vi "LCWP950 Signal Acquisition.vi"(0 "VISA resource name in":refnum<visa-resource-name>="VICP::172.25.1.26", 3 "Query Instrument?":bool=TRUE, 5 "error in (no error)":errorcluster) -> (14 "VISA resource name out":refnum<visa-resource-name>, 19 "error out":errorcluster)   [LabVIEW 2012]
uses:
  <vilib>/Instr/_visa.llb/VISA Open Access Mode.ctl
panel:
  in  "?":T1(tab)
  in  "Save Folder":path=path "C:/TEST"
  out "Run Count":i32
  in  "N Loops":i32
  out "C1:\nC2:\n   t:":string
  in  "Byte count":u32=160800
  out "Identity":string
  # "Neil McBlane 2016"
  # "NOTE: VISA Read byte count will need increased for reading >400 points - e.g. try\n320800 for 800 points. For n points: 4 bytes per point, n+2 points recorded 100 times."
  # "NOTE: code 1073676294 is not an error - it indicates the buffer has been read in its entirety"
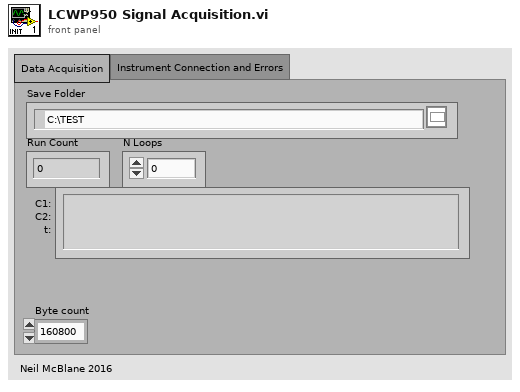
[diagram p1: front panel]
types:
  T1 = enum32{"Data Acquisition", "Instrument Connection and Errors"}
  T2 = typedef "VISA Open Access Mode.ctl" = u32
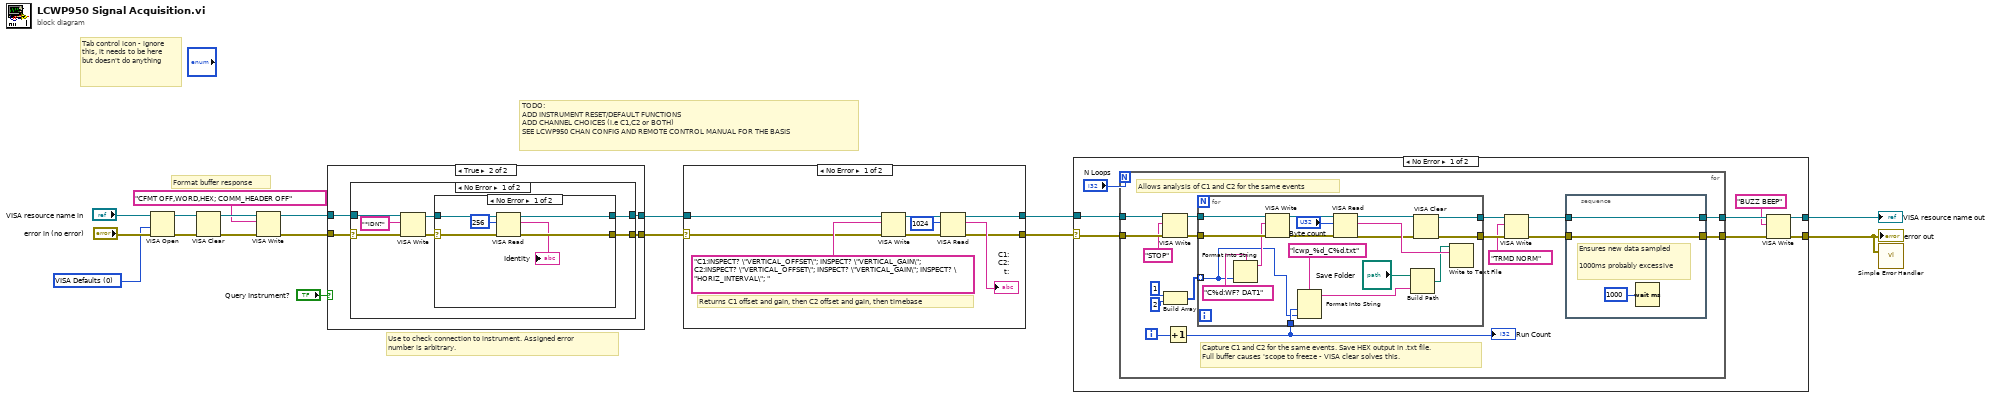
[diagram p0: block diagram]
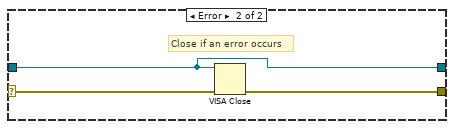
[diagram p2: hidden frame]
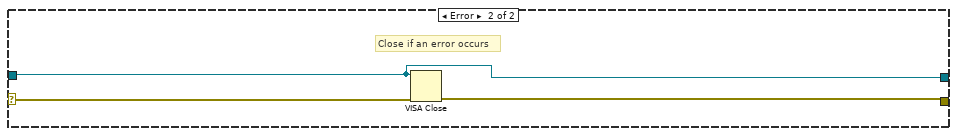
[diagram p3: hidden frame]
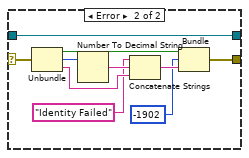
[diagram p5: hidden frame]
diagram:
  w15 = T2 0 items=["VISA Defaults"=0, "Exclusive Lock"=1, "Load Configured Settings"=4] ("Access Mode")
  # "Tab control icon - ignore this, it needs to be here but doesn't do anything"
  # "Use to check connection to instrument. Assigned error number is arbitrary."
  # "Format buffer response"
  # "TODO: \nADD INSTRUMENT RESET/DEFAULT FUNCTIONS\nADD CHANNEL CHOICES (i.e C1,C2 or BOTH)\nSEE LCWP950 CHAN CONFIG AND REMOTE CONTROL MANUAL FOR THE BASIS"
  n1 = VISA Open(access mode=w15, error in (no error)="error in (no error)", VISA resource name="VISA resource name in") -> (VISA resource name=w14:refnum<visa-resource-name>, error out=w13:errorcluster)  [unwired: 2 in]
  n2 = VISA Clear(VISA resource name=w14, error in (no error)=w13) -> (VISA resource name out=w9:refnum<visa-resource-name>, error out=w8:errorcluster)
  n3 = VISA Write(VISA resource name=w9, write buffer="CFMT OFF,WORD,HEX; COMM_HEADER OFF", error in (no error)=w8) -> (VISA resource name out=w6:refnum<visa-resource-name>, error out=w7:errorcluster)  [unwired: 1 out]
  n4 = case shown="True" "Query Instrument?" {
    tunnel: w6 -> [w19 w23]
    tunnel: w7 -> [w18 w22]
    tunnel: [w18 w21] -> w1
    tunnel: [w19 w20] -> w4
    frame False {
    }
    frame True {
      n5 = case shown="No Error" w22 {
        selector: w22 -> [w28 w48]
        tunnel: w23 -> [w29 w47]
        tunnel: [w24 w48] -> w21
        tunnel: [w26 w47] -> w20
        frame No Error {
          n6 = VISA Write(VISA resource name=w29, write buffer="*IDN?", error in (no error)=w28) -> (VISA resource name out=w27:refnum<visa-resource-name>, error out=w25:errorcluster)  [unwired: 1 out]
          n7 = case shown="No Error" w25 {
            selector: w25 -> [w36 w45]
            tunnel: w27 -> [w35 w46]
            tunnel: [w34 w46] -> w26
            tunnel: [w33 w43] -> w24
            frame No Error {
              n8 = VISA Read(VISA resource name=w35, byte count=u32 256, error in (no error)=w36) -> (VISA resource name out=w34:refnum<visa-resource-name>, read buffer=→"Identity":string, error out=w33:errorcluster)  [unwired: 1 out]
            }
            frame Error {
              n9 = Unbundle(w45) -> ("status"=w44:bool, "code"=w42:i32, "source"=w39:string)
              n10 = Number To Decimal String(number=w42) -> (decimal integer string=w41:string)  [unwired: 1 in]
              n11 = Concatenate Strings("Identity Failed", w41, w39) -> (w40:string)
              n12 = Bundle("status"=w44, -1902, w40) -> (w43:cluster{"status":bool, i32, string})  [unwired: 1 in]
            }
          }
        }
        frame Error {
        }
      }
    }
  }
  n13 = case shown="No Error" w1 {
    selector: w1 -> [w49 w60]
    tunnel: w4 -> [w52 w58]
    tunnel: [w51 w58] -> w3
    tunnel: [w50 w59] -> w2
    frame No Error {
      # "Returns C1 offset and gain, then C2 offset and gain, then timebase"
      n14 = VISA Write(VISA resource name=w52, write buffer="C1:INSPECT? \"VERTICAL_OFFSET\"; INSPECT? \"VERTICAL_GAIN\"; C2:INSPECT? \"VERTICAL_OFFSET\"; INSPECT? \"VERTICAL_GAIN\"; INSPECT? \"HORIZ_INTERVAL\"; ", error in (no error)=w49) -> (VISA resource name out=w54:refnum<visa-resource-name>, error out=w55:errorcluster)  [unwired: 1 out]
      n15 = VISA Read(VISA resource name=w54, byte count=u32 1024, error in (no error)=w55) -> (VISA resource name out=w51:refnum<visa-resource-name>, read buffer=→"C1:\nC2:\n   t:":string, error out=w50:errorcluster)  [unwired: 1 out]
    }
    frame Error {
      # "Close if an error occurs"
      n16 = VISA Close(VISA resource name=w58, error in (no error)=w60) -> (error out=w59:errorcluster)
    }
  }
  n17 = case shown="No Error" w2 {
    selector: w2 -> [w67 w109]
    tunnel: [w63 w108] -> w10
    tunnel: w3 -> [w68 w107]
    tunnel: [w65 w107] -> w11
    frame No Error {
      n18 = for {
        N: "N Loops" -> [_]
        tunnel: w68 -> [w84]
        tunnel: w67 -> [w85]
        tunnel: [w71] -> w64
        tunnel: [w69] -> w66
        i -> [w74]
        # "Allows analysis of C1 and C2 for the same events"
        # "Capture C1 and C2 for the same events. Save HEX output in .txt file. \nFull buffer causes 'scope to freeze - VISA clear solves this."
        n19 = VISA Write(VISA resource name=w84, write buffer="STOP", error in (no error)=w85) -> (VISA resource name out=w82:refnum<visa-resource-name>, error out=w81:errorcluster)  [unwired: 1 out]
        n20 = Build Array(1, 2) -> (w80:i32[])
        n21 = Increment(x=w74) -> (x+1=w73:i32)
        "Run Count" <- w73
        n22 = for {
          tunnel: w82 -> [w106]
          tunnel: w81 -> [w105]
          tunnel: w80 -> [w96] mode=indexing
          tunnel: w73 -> [w97]
          tunnel: [w92] -> w77
          tunnel: [w91] -> w76
          n23 = Format Into String(format string="C%d:WF? DAT1", w96) -> (resulting string=w101:string)  [unwired: 2 in, 1 out]
          n24 = VISA Write(VISA resource name=w106, write buffer=w101, error in (no error)=w105) -> (VISA resource name out=w103:refnum<visa-resource-name>, error out=w104:errorcluster)  [unwired: 1 out]
          n25 = Format Into String(format string="lcwp_%d_C%d.txt", w97, w96) -> (resulting string=w89:string)  [unwired: 2 in, 1 out]
          n26 = VISA Read(VISA resource name=w103, byte count="Byte count", error in (no error)=w104) -> (VISA resource name out=w93:refnum<visa-resource-name>, read buffer=w98:string, error out=w90:errorcluster)  [unwired: 1 out]
          n27 = Build Path(base path="Save Folder", name or relative path=w89) -> (appended path=w94:path)
          n28 = VISA Clear(VISA resource name=w93, error in (no error)=w90) -> (VISA resource name out=w92:refnum<visa-resource-name>, error out=w91:errorcluster)
          n29 = Write to Text File(file (use dialog)=w94, text=w98) -> ()  [unwired: 2 in, 3 out]
        }
        n30 = VISA Write(VISA resource name=w77, write buffer="TRMD NORM", error in (no error)=w76) -> (VISA resource name out=w70:refnum<visa-resource-name>, error out=w72:errorcluster)  [unwired: 1 out]
        n31 = stacked-sequence {
          tunnel: w72 -> [w87]
          tunnel: [w87] -> w71
          tunnel: w70 -> [w86]
          tunnel: [w86] -> w69
          frame #0 {
            # "Ensures new data sampled\n\n1000ms probably excessive"
            n32 = Wait (ms)(milliseconds to wait=u32 1000) -> ()  [unwired: 1 out]
          }
        }
      }
      n33 = VISA Write(VISA resource name=w66, write buffer="BUZZ BEEP", error in (no error)=w64) -> (VISA resource name out=w65:refnum<visa-resource-name>, error out=w63:errorcluster)  [unwired: 1 out]
    }
    frame Error {
      # "Close if an error occurs"
      n34 = VISA Close(VISA resource name=w107, error in (no error)=w109) -> (error out=w108:errorcluster)
    }
  }
  "VISA resource name out" <- w11
  "error out" <- w10
  n35 = call <vilib>:"Simple Error Handler.vi"("error in (no error)"=w10) -> ()  [unwired: 4 in, 5 out]
